vi "Test Rounded Corner VI.vi"() -> ()   [LabVIEW 2013]
panel:
  in  "Tab Control":enum32{"Page 1", "Page 2"}(tab)
  in  "Numeric":dbl
  in  "Numeric 2":dbl
  in  "Numeric 3":dbl
  in  "Numeric 4":dbl
  in  "String":string
  in  "Listbox":i32(listbox)
  in  "Exit":bool
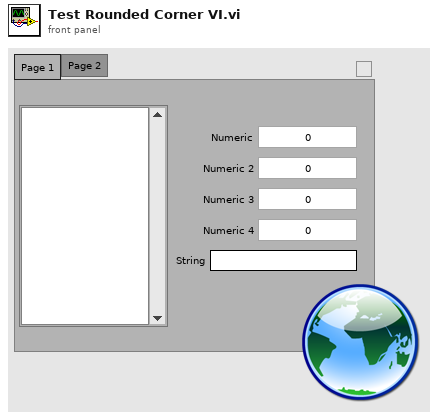
[diagram p1: front panel]
types:
  T1 = typedef "LVPoint32TypeDef.ctl" = cluster{"Horizontal":i32, "Vertical":i32}
  T2 = typedef "LVPositionTypeDef.ctl" = cluster{"Left":i32, "Top":i32}
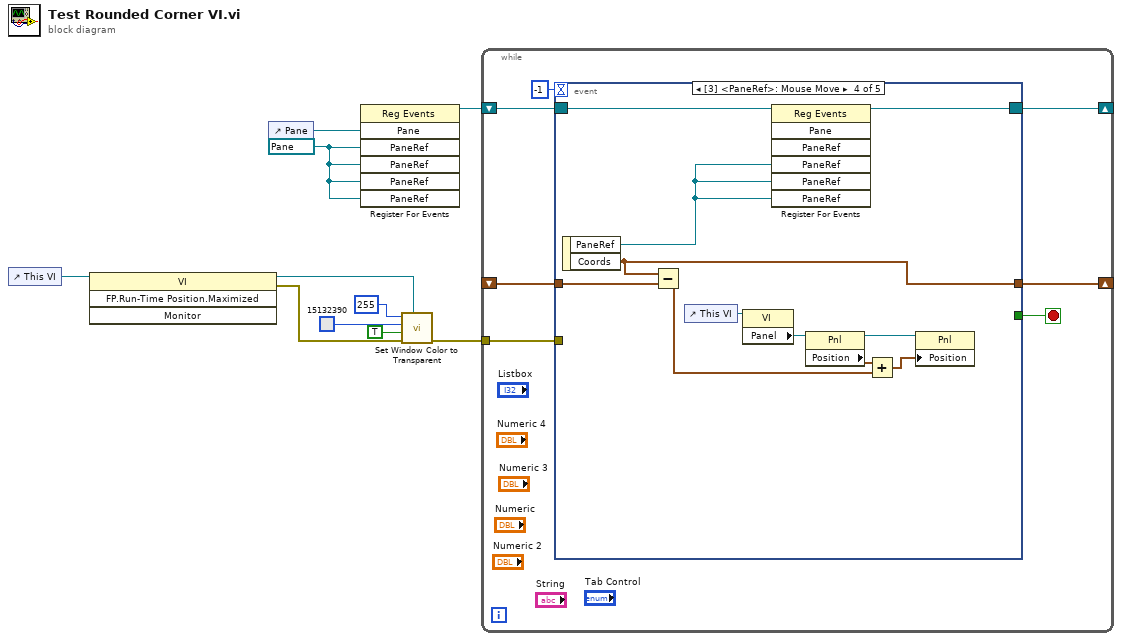
[diagram p0: block diagram]
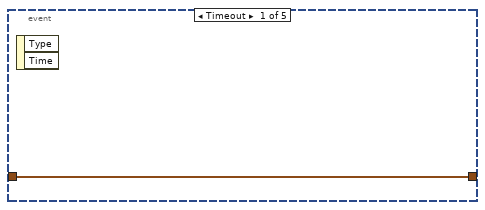
[diagram p2: hidden frame]
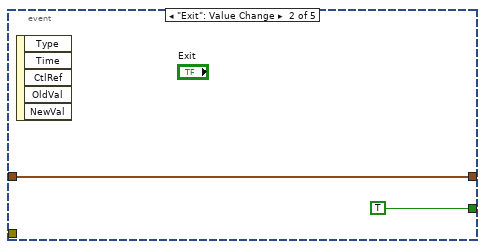
[diagram p3: hidden frame]
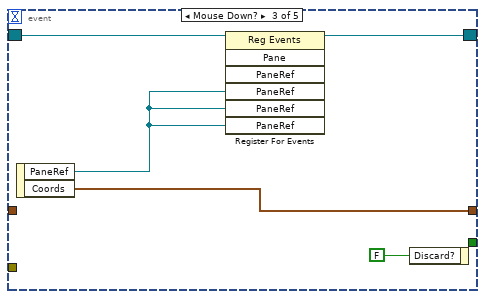
[diagram p4: hidden frame]
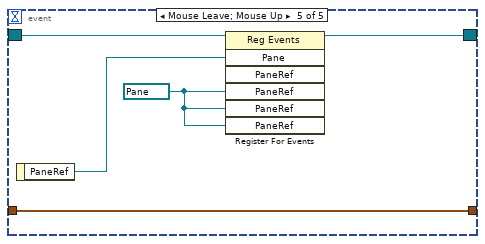
[diagram p5: hidden frame]
diagram:
  w6 = refnum<vi> refnum ("PaneRef")
  n1 = control-ref of="This VI"() -> (w4:refnum<vi>)
  n2 = invoke class="VI" method="FP.Run-Time Position.Maximized"(reference=w4) -> (reference out=w2:refnum<vi>, error out=w3:errorcluster)  [unwired: 3 in, 2 out]
  n3 = control-ref of="Pane"() -> (w5:refnum<vi>)
  n4 = register-events(w5, w6, w6, w6, w6) -> (reference out=w7:refnum<event-registration>)  [unwired: 2 in, 1 out]
  n5 = call "Set Window Color to Transparent.vi"("Calling VI's reference"=w2, "error in (no error)"=w3, "Activate"=TRUE, "Color to Replace"=u32 15132390, "Factor"=u8 255) -> ("error out"=w1:errorcluster)  [unwired: 3 in]
  n6 = while {
    tunnel: w1 -> [w16]
    shift-right: [w13] -> _
    shift-left: w7 -> [w14]
    shift-right: [w12] -> _
    shift-left: _ -> [w11]
    stop <- w15 stop-if-true
    n7 = event shown="[3] <PaneRef>: Mouse Move" {
      selector: w14 -> [_ _ w25 w36 w41]
      dyn-events: [_ _ w24 w35 w40] -> w13
      timeout: -1 -> [_ _ _ _ _]
      tunnel: w16 -> [_ _ _ _ _]
      tunnel: [_ TRUE _ _ _] -> w15
      tunnel: [w18 w19 w21 w33 w39] -> w12
      tunnel: w11 -> [w18 w19 _ w32 w39]
      event Timeout {
        n8 = event-data() -> ()  [unwired: 1 in, 2 out]
      }
      event "Exit": Value Change {
        n9 = event-data() -> ()  [unwired: 1 in, 5 out]
      }
      event Mouse Down? {
        n10 = event-data() -> ("PaneRef"=w22:refnum<vi>, "Coords"=w21:T1)  [unwired: 1 in]
        n11 = register-events(reference=w25, w22, w22, w22) -> (reference out=w24:refnum<event-registration>)  [unwired: 3 in, 1 out]
        n12 = event-data("Discard?"=FALSE) -> ()  [unwired: 1 in, 1 out]
      }
      event Mouse Move {
        n13 = event-data() -> ("PaneRef"=w34:refnum<vi>, "Coords"=w33:T1)  [unwired: 1 in]
        n14 = Subtract(x=w33, y=w32) -> (x-y=w27:T1)
        n15 = control-ref of="This VI"() -> (w31:refnum<vi>)
        n16 = property class="VI"(reference=w31) -> ("Panel"=w30:refnum<vi>)  [unwired: 1 in, 2 out]
        n17 = register-events(reference=w36, w34, w34, w34) -> (reference out=w35:refnum<event-registration>)  [unwired: 3 in, 1 out]
        n18 = property class="Pnl"(reference=w30) -> (reference out=w29:refnum<vi>, "Position"=w28:T2)  [unwired: 1 in, 1 out]
        n19 = Add(x=w28, y=w27) -> (x+y=w26:T2)
        n20 = property class="Pnl"(reference=w29, "Position"=w26) -> ()  [unwired: 1 in, 2 out]
      }
      event Mouse Leave; Mouse Up {
        w38 = refnum<vi> refnum ("PaneRef")
        n21 = event-data() -> ("PaneRef"=w37:refnum<vi>)  [unwired: 1 in]
        n22 = register-events(reference=w41, w37, w38, w38, w38) -> (reference out=w40:refnum<event-registration>)  [unwired: 2 in, 1 out]
      }
    }
  }
